vi "Robot Radii.vi"() -> ()   [LabVIEW 2011]
panel:
  in  "Robot Radii":cluster{"Short":dbl, "Long":dbl}={"Short"=10.0, "Long"=13.625}
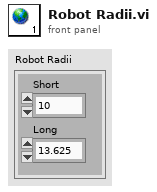
[diagram p1: front panel]
diagram:
